vi "Format Weather Data.vi"(8 "Error In":errorcluster, 11 "Display Manager In":refnum<class "Display Manager.lvclass">) -> (0 "Error Out":errorcluster, 2 "Weather String":string, 3 "Display Manager Out":refnum<class "Display Manager.lvclass">)   [LabVIEW 2021, in "Display Manager.lvclass"]
uses:
  Display Manager.lvclass
  Controls/Weather FGV Method.ctl
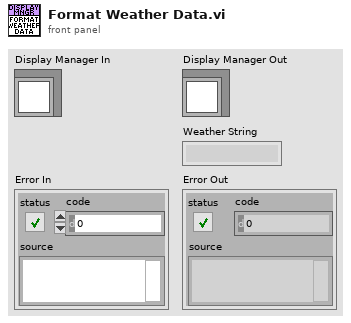
[diagram p1: front panel]
types:
  T1 = typedef "Display Manager.lvclass/Weather FGV Method.ctl" = enum16{"Initialize", "Query Weather"}
  T2 = typedef "Open Weather Session.lvclass/Weather Data.ctl" = cluster{"Timezone":string, "Timezone Offset":dbl, "Weather Sample Data":T3}
  T3 = typedef "Open Weather Session.lvclass/Weather Sample Data.ctl" = cluster{"Current Time":timestamp, "Sunrise":timestamp, "Sunset":timestamp, "Temperature (C)":dbl, "Feels Like Temperature (C)":dbl, "Atmospheric Pressure (hPa)":dbl, "Humidity (%)":dbl, "Dew Point (C)":dbl, "Cloudiness (%)":dbl, "UV Index":dbl, "Visibility (m)":dbl, "Wind Speed (m/s)":dbl, "Wind Direction (degrees)":dbl, "Weather Data":T4}
  T4 = typedef "Open Weather Session.lvclass/Weather Description Data.ctl" = cluster{"main":string, "description":string}
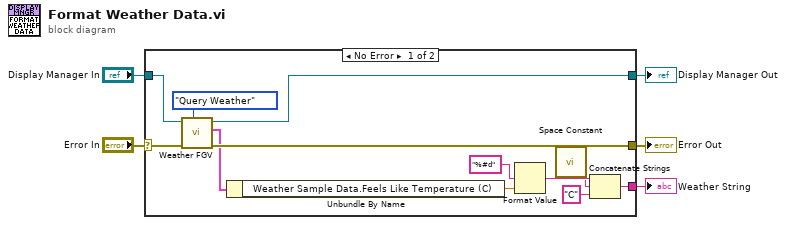
[diagram p0: block diagram]
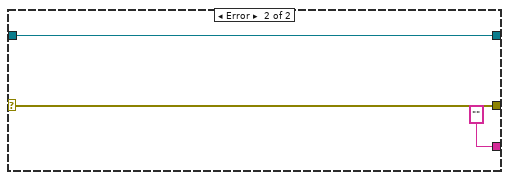
[diagram p2: hidden frame]
diagram:
  n1 = case shown="No Error" "Error In" {
    selector: "Error In" -> [w17 w20]
    tunnel: [w13 w20] -> w4
    tunnel: "Display Manager In" -> [w8 w19]
    tunnel: [w6 w19] -> w2
    tunnel: [w10 ""] -> w1
    frame No Error {
      n2 = call "Weather FGV.vi"("Weather FGV Method"=Weather_FGV_Method."Query Weather", "Error In"=w17, "Display Manager In"=w8) -> ("Error Out"=w13:errorcluster, "Weather Data"=w7:T2, "Display Manager Out"=w6:refnum<class "Display Manager.lvclass">)  [unwired: 6 in]
      n3 = Unbundle By Name(w7) -> ("Weather Sample Data.Feels Like Temperature (C)"=w16:dbl)
      n4 = Format Value(format string="%#d", value (0)=w16) -> (output string=w14:string)  [unwired: 1 in]
      n5 = call <vilib>:"Space Constant.vi"() -> ("String"=w12:string)
      n6 = Concatenate Strings(w14, w12, "C" ("string")) -> (w10:string)
    }
    frame Error {
    }
  }
  "Display Manager Out" <- w2
  "Error Out" <- w4
  "Weather String" <- w1
